vi "Global.vi"() -> ()   [LabVIEW 2017]
panel:
  in  "Names":string[](array[string])
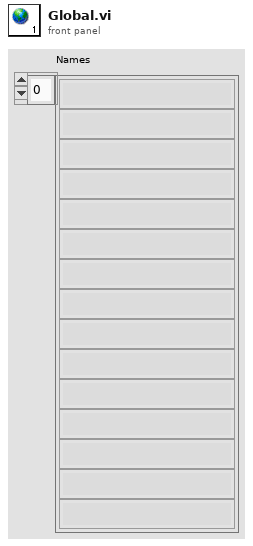
[diagram p1: front panel]
diagram:
